vi "TableReceiverTactic.vi"(7 "Firstcall?":bool=TRUE, 8 "error in (no error)":errorcluster, 9 "Game in":refnum<class "Game.lvclass">, 10 "Robot":refnum<class "Robot.lvclass">, 11 "TableReceiverTactic in":refnum<class "TableReceiverTactic.lvclass">) -> (0 "error out":errorcluster, 2 "Robot out":refnum<class "Robot.lvclass">, 3 "TableReceiverTactic out":refnum<class "TableReceiverTactic.lvclass">)   [LabVIEW 2020, in "TableReceiverTactic.lvclass"]
uses:
  TableReceiverTactic.lvclass
  Robot_class/Robot.lvclass
  Game_class/Game.lvclass
  Robot_class/tactics.ctl
  Tactic_class/Tactic.lvclass/Tactic.ctl
  Game_class/Game.lvclass/Game.ctl
  Skillbook_class/Skillbook.lvclass/Skillbook.ctl
  Robot_class/Robot.lvclass/Robot.ctl
  TableReceiverTactic.lvclass/TableReceiverTactic.ctl
  Skillbook_class/Read TableReceiverGoToSkill.vi
  Game_class/Read Utilities.lvclass.vi
  Game_class/Read BallRef.vi
  Skillbook_class/Read HaltSkill.vi
  Robot_class/Write dest_orientation.vi
  Game_class/Read OffensiveTeam.vi
  Game_class/Read FieldRef.vi
  Tactic_class/Read Skillbook.vi
  Write States.vi
  Robot_class/Write tactic.vi
  Utilities_class/Utilities.lvclass
  Ally_class/Ally.lvclass
  Ball_class/Ball.lvclass
  Field_class/Field.lvclass
  Skillbook_class/Skillbook.lvclass
  TableReceiverGoToSkill_class/TableReceiverGoToSkill.lvclass
  HaltSkill_class/HaltSkill.lvclass
panel:
  out "x .or. y?":bool
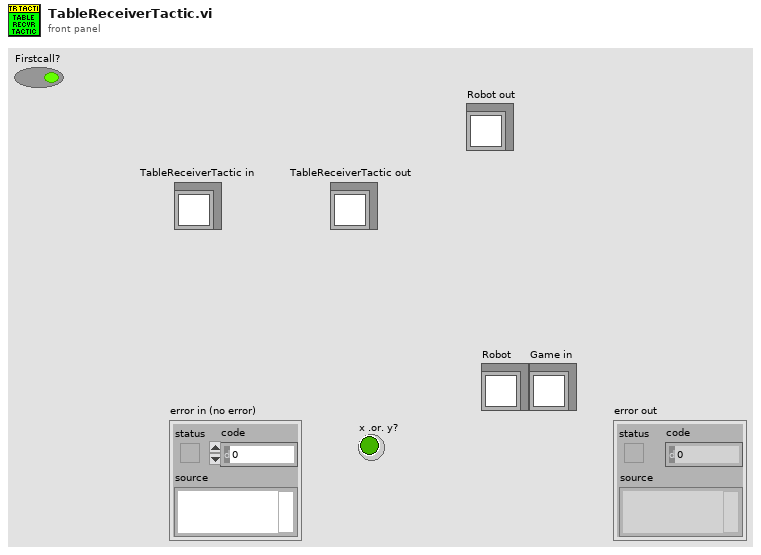
[diagram p1: front panel]
types:
  T1 = typedef "tactics.ctl" = enum16{"5Robots", "BallPlacementEnemy", "ReceivePassInFuturePoint", "Roller", "PrepareRollToPassRollerGoTo", "PrepareRollToPassReceiverGoTo", "WaitRoll", "PositionToRoll", "PenaltyAttacker", "PassObserver", "PenaltyDefense", "TableReceiverTactic", "Test", "DefendGoal", "Marker", "FollowAttacker", "DefendArea", "Shoot", "AttackerAimGoal", "AttackerBallOutOfField", "AttackerBlock", "AttackerStop", "Duelist", "Halt", "ZigZag", "GoTo", "Timeout", "KickToBestRobot", "KickToPassReceiver", "PositionToReceivePass", "WaitPass"}
  T2 = typedef "KickToPassReceiverTacticStates.ctl" = enum16{"Halt", "GoToReceiveTable", "KickToPassReceiver", "WaitPass", "Exit"}
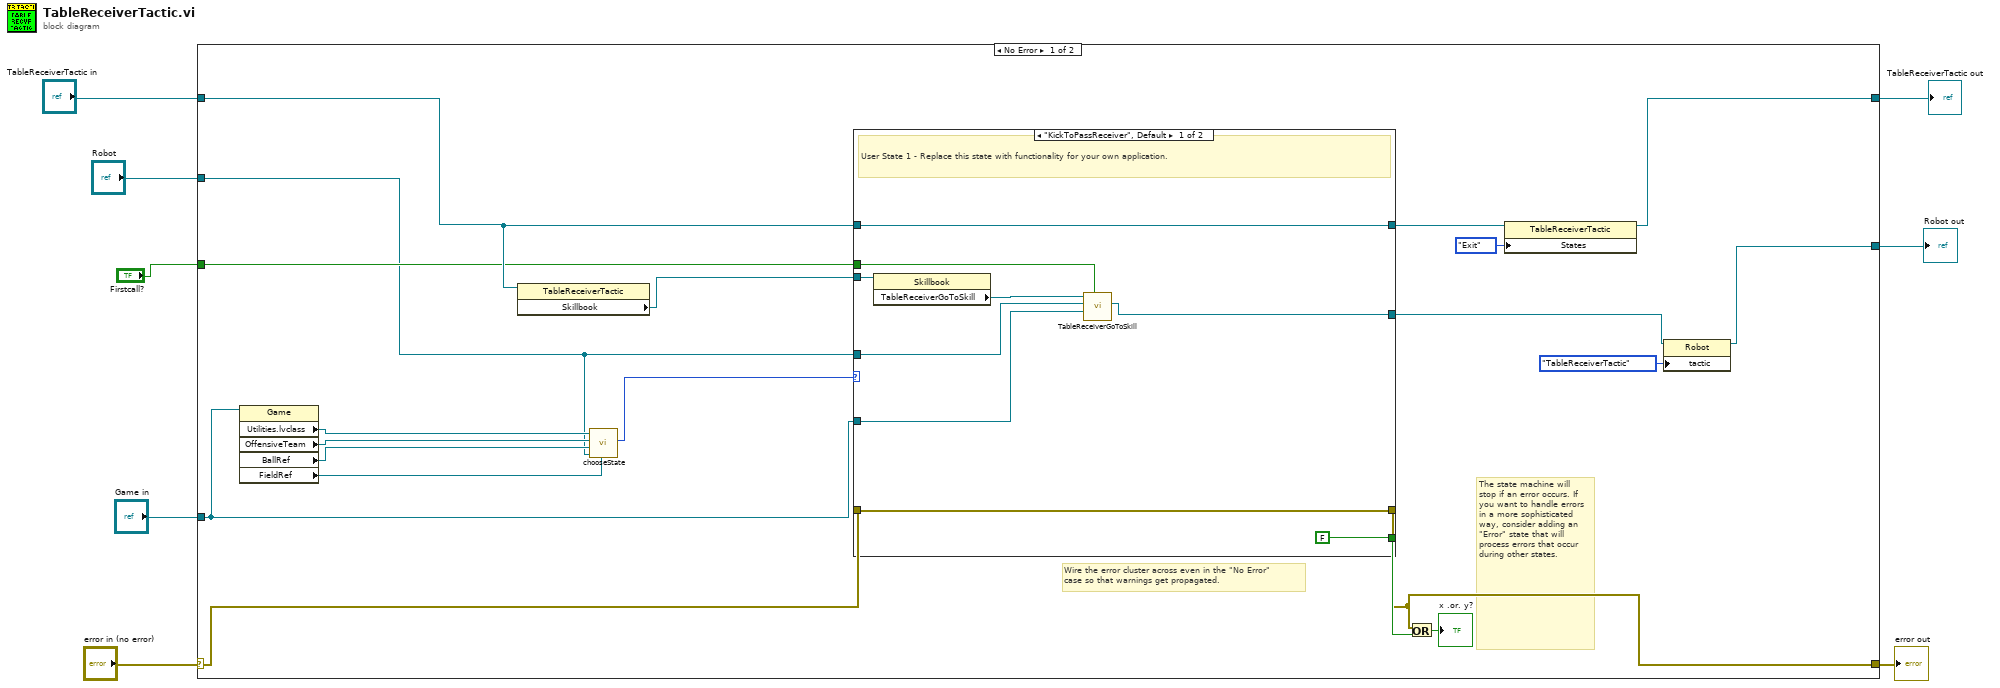
[diagram p0: block diagram]
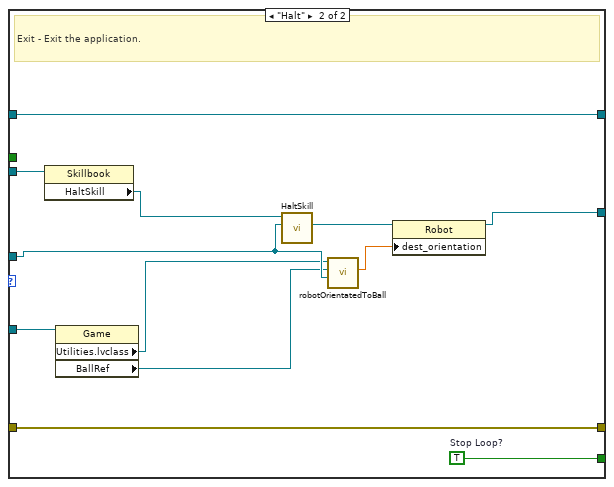
[diagram p2: hidden frame]
diagram:
  n1 = case shown="No Error" "error in (no error)" {
    selector: "error in (no error)" -> [w24 w52]
    tunnel: [w23 w52] -> w7
    tunnel: [w21 w51] -> w2
    tunnel: "TableReceiverTactic in" -> [w22 w51]
    tunnel: "Robot" -> [w10 w50]
    tunnel: "Game in" -> [w16 _]
    tunnel: [w19 w50] -> w4
    tunnel: "Firstcall?" -> [w13 _]
    frame No Error {
      # "The state machine will stop if an error occurs. If you want to handle errors in a more sophisticated way, consider adding an \"Error\" state that will process errors that occur during other states."
      # "Wire the error cluster across even in the \"No Error\"\ncase so that warnings get propagated."
      n2 = property class="Game"(reference=w16) -> ("Utilities.lvclass"=w18:refnum<class "Utilities.lvclass">, "OffensiveTeam"=w17:refnum<class "Ally.lvclass">, "BallRef"=w12:refnum<class "Ball.lvclass">, "FieldRef"=w9:refnum<class "Field.lvclass">)  [unwired: 1 in, 2 out]
      n3 = property class="TableReceiverTactic"(reference=w22) -> ("Skillbook"=w26:refnum<class "Skillbook.lvclass">)  [unwired: 1 in, 2 out]
      n4 = call "chooseState.vi"("FieldRef"=w9, "Robot"=w10, "BallRef"=w12, "OffensiveTeam"=w17, "Utilities in"=w18) -> ("state"=w11:T2)  [unwired: 6 in]
      n5 = case shown="\"KickToPassReceiver\", Default" w11 {
        tunnel: [FALSE ("Stop Loop?") w49] -> w28
        tunnel: w24 -> [w36 w48]
        tunnel: [w36 w48] -> w23
        tunnel: w26 -> [w35 w46]
        tunnel: w10 -> [w31 w41]
        tunnel: [w32 w43] -> w20
        tunnel: [w34 w47] -> w25
        tunnel: w22 -> [w34 w47]
        tunnel: w16 -> [w30 w40]
        tunnel: w13 -> [w29 _]
        frame "KickToPassReceiver", Default {
          # "User State 1 - Replace this state with functionality for your own application."
          n6 = property class="Skillbook"(reference=w35) -> ("TableReceiverGoToSkill"=w33:refnum<class "TableReceiverGoToSkill.lvclass">)  [unwired: 1 in, 2 out]
          n7 = call "TableReceiverGoToSkill.vi"("Firstcall?"=w29, "Game"=w30, "Robot in"=w31, "TableReceiverGoToSkill in"=w33) -> ("Robot out"=w32:refnum<class "Robot.lvclass">)  [unwired: 5 in, 2 out]
        }
        frame "Halt" {
          w49 = TRUE  # Stop Loop?
          # "Exit - Exit the application."
          n8 = property class="Skillbook"(reference=w46) -> ("HaltSkill"=w45:refnum<class "HaltSkill.lvclass">)  [unwired: 1 in, 2 out]
          n9 = property class="Game"(reference=w40) -> ("Utilities.lvclass"=w38:refnum<class "Utilities.lvclass">, "BallRef"=w39:refnum<class "Ball.lvclass">)  [unwired: 1 in, 2 out]
          n10 = call-dynamic "HaltSkill.vi"("Robot"=w41, "HaltSkill in"=w45) -> ("Robot out"=w44:refnum<class "Robot.lvclass">)  [unwired: 7 in, 2 out]
          n11 = call "robotOrientatedToBall.vi"("Robot"=w41, "BallRef"=w39, "Utilities in"=w38) -> ("Orientation"=w42:dbl)  [unwired: 6 in, 2 out]
          n12 = property class="Robot"(reference=w44, "dest_orientation"=w42) -> (reference out=w43:refnum<class "Robot.lvclass">)  [unwired: 1 in, 1 out]
        }
      }
      n13 = Or(x=w23, y=w28) -> (x .or. y?=→"x .or. y?":bool)
      n14 = property class="TableReceiverTactic"(reference=w25, "States"=enum16{"Halt", "Exit", "GoTo"}."Exit") -> (reference out=w21:refnum<class "TableReceiverTactic.lvclass">)  [unwired: 1 in, 1 out]
      n15 = property class="Robot"(reference=w20, "tactic"=tactics."TableReceiverTactic") -> (reference out=w19:refnum<class "Robot.lvclass">)  [unwired: 1 in, 1 out]
    }
    frame Error {
    }
  }
  "error out" <- w7
  "Robot out" <- w4
  "TableReceiverTactic out" <- w2
